vi "获取最新数据.vi"(8 "error in (no error)":errorcluster caption="错误输入（无错误）", 10 "table":string, 11 "database":string) -> (0 "error out":errorcluster caption="错误输出", 2 "data":string[][](table), 3 "子数组":variant[](array[variant]))   [LabVIEW 2016]
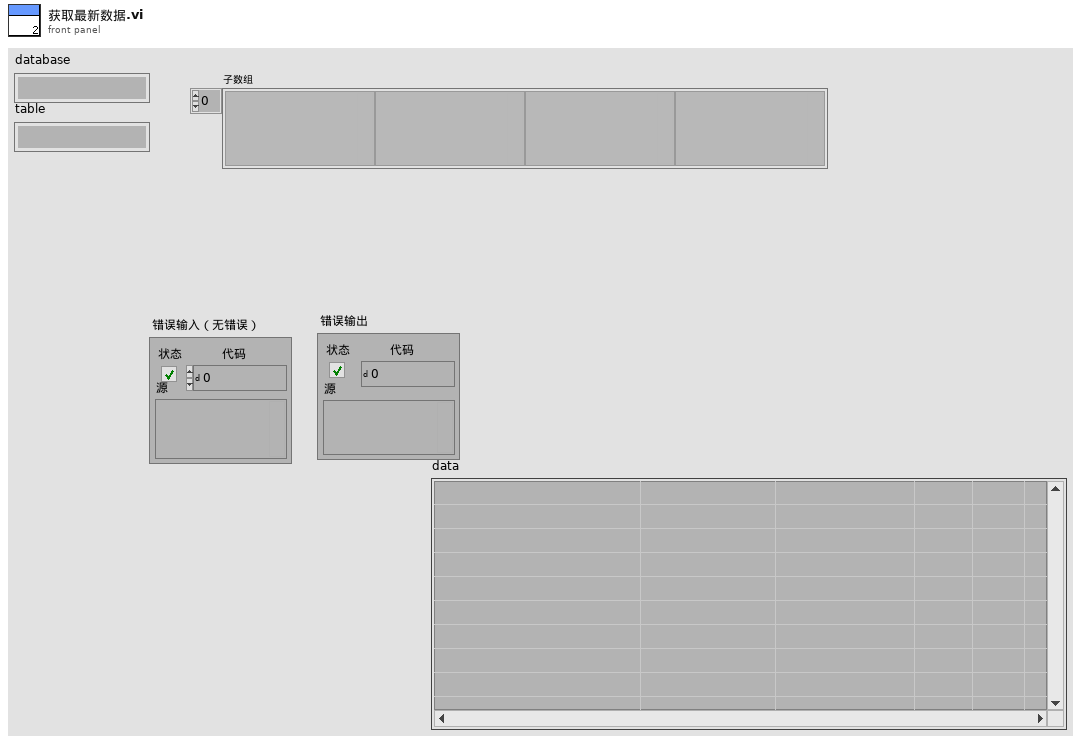
[diagram p1: front panel]
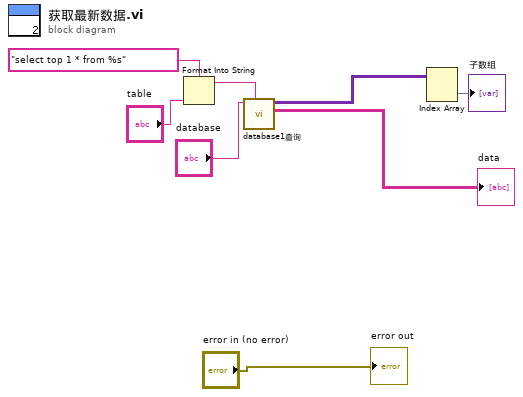
[diagram p0: block diagram]
diagram:
  n1 = Format Into String(format string="select top 1 * from %s" ("格式字符串"), "table") -> (resulting string=w7:string)  [unwired: 2 in, 1 out]
  n2 = call "database1查询.vi"("SQL query"=w7, "database"="database") -> ("data"=→"data":string[][], "recordset data"=w4:variant[][])  [unwired: 7 in, 1 out]
  n3 = Index Array(array=w4) -> (element=→"子数组":variant[])  [unwired: 2 in]
  "error out" <- "error in (no error)"
